vi "EMD8216 counter mask set.vi"(9 "channel":u8, 10 "port":u8, 11 "CardID":u32) -> (3 "error_code":u32)   [LabVIEW 2009, in "EMD8216_64.lvlib"]
doc: "EMD8216Status EMD8216_counter_mask_set(u32 CardID,u8 port,u8 channel);"
uses:
  EMD8216_64.lvlib
  <userlib>/EMD8216_64/EMD8216_64.dll
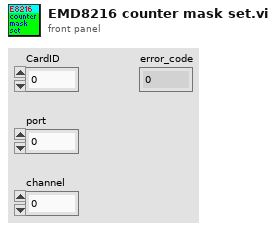
[diagram p1: front panel]
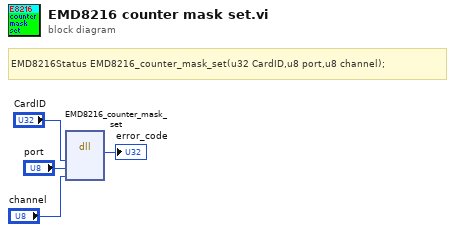
[diagram p0: block diagram]
diagram:
  # "EMD8216Status EMD8216_counter_mask_set(u32 CardID,u8 port,u8 channel);"
  n1 = dll-call lib="C:/Program Files/National Instruments/LabVIEW 2017/user.lib/EMD8216_64/EMD8216_64.*" fn="EMD8216_counter_mask_set"("CardID"="CardID", "port"="port", "channel"="channel") -> (→"error_code":u32)  [unwired: 6 in, 2 out]
